vi "Handle Error.vi"(8 "error in (no error)":errorcluster, 11 "SignalProcessing in":refnum<class "SignalProcessing.lvclass">) -> (0 "error out":errorcluster, 2 "stop actor?":bool=TRUE, 3 "SignalProcessing out":refnum<class "SignalProcessing.lvclass">)   [LabVIEW 2019, in "SignalProcessing.lvlib" / "SignalProcessing.lvclass"]
doc: "(<B>Filename</B>: Actor Framework.lvlib:Actor.lvclass:Handle Error.vi)\n\nDefines how the actor handles an error that occurred while processing a message. By default, this method does nothing except stop the actor."
uses:
  SignalProcessing.lvclass
  <vilib>/NI/Event Source Actor/Event Source/Event Source/Event Source.lvclass
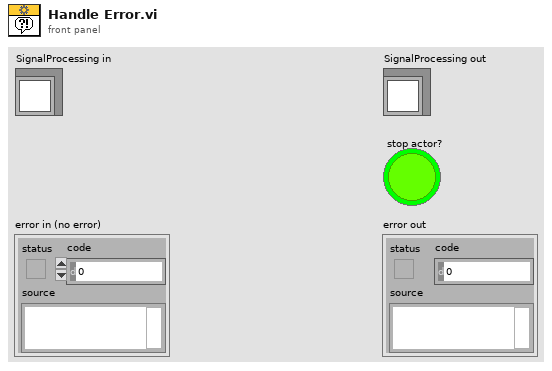
[diagram p1: front panel]
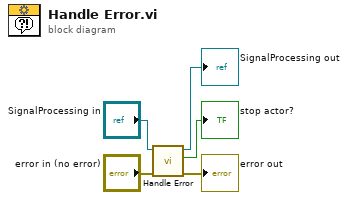
[diagram p0: block diagram]
diagram:
  n1 = call-parent "Handle Error.vi"("error in (no error)"="error in (no error)", "Actor in"="SignalProcessing in") -> ("error out"=→"error out":errorcluster, "stop actor?"=→"stop actor?":bool, "Actor out"=→"SignalProcessing out":refnum<class "SignalProcessing.lvclass">)  [unwired: 7 in]
